vi "close hardware connections.vi"(11 "Template in":refnum<class "Template.lvclass">) -> (3 "Template out":refnum<class "Template.lvclass">)   [LabVIEW 2020, in "Template.lvlib" / "Template.lvclass"]
doc: "Executes any hardware closing procedure here.\nThis vi is called in the Stop Core override of the Actor Framework overrides."
uses:
  Template.lvclass
  Template.lvclass/Template.ctl
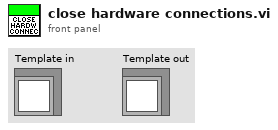
[diagram p1: front panel]
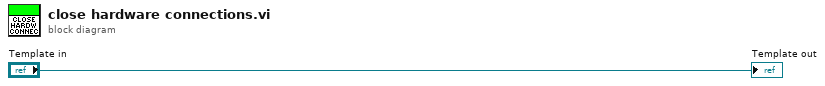
[diagram p0: block diagram]
diagram:
  "Template out" <- "Template in"
